vi "DisplayPanel.vi"() -> ()   [LabVIEW 2013]
uses:
  MvLVLib/MvCameraControl.lvlib
panel:
  in  "TimerTriggerActivation":u16(ring) items=["RisingEdge", "FallingEdge", "AnyEdge", "LevelHigh", "LevelLow"]
  in  "TimerTriggerSoftware":bool
  in  "TimerTriggerSource":u16(ring) items=["Off", "OptoCoupledInput0", "OptoCoupledInput1", "OptoCoupledInput2", "OptoCoupledInput3", "RS422diffInput0", "RS422diffInput1", "RS422diffInput2", "RS422diffInput3", "TTLInput0", "TTLInput1", "TTLInput2", "TTLInput3", "Timer0Active", "Timer1Active", "Timer2Active", "Timer3Active", "Encoder0", "Encoder1", "SoftwareSignal0", "Continuous"]
  in  "TimerFrequency":u32
  in  "TimerDelay":u32
  in  "TimerDuration":u32
  in  "TimerSelector":u16(ring) items=["Timer0", "Timer1", "Timer2", "Timer3"]
  in  "Interface List":u16(ring)
  out "handle":u64 format="%x"
  in  "Close Interface":bool
  in  "Open Interface":bool
  in  "Enum Interface":bool
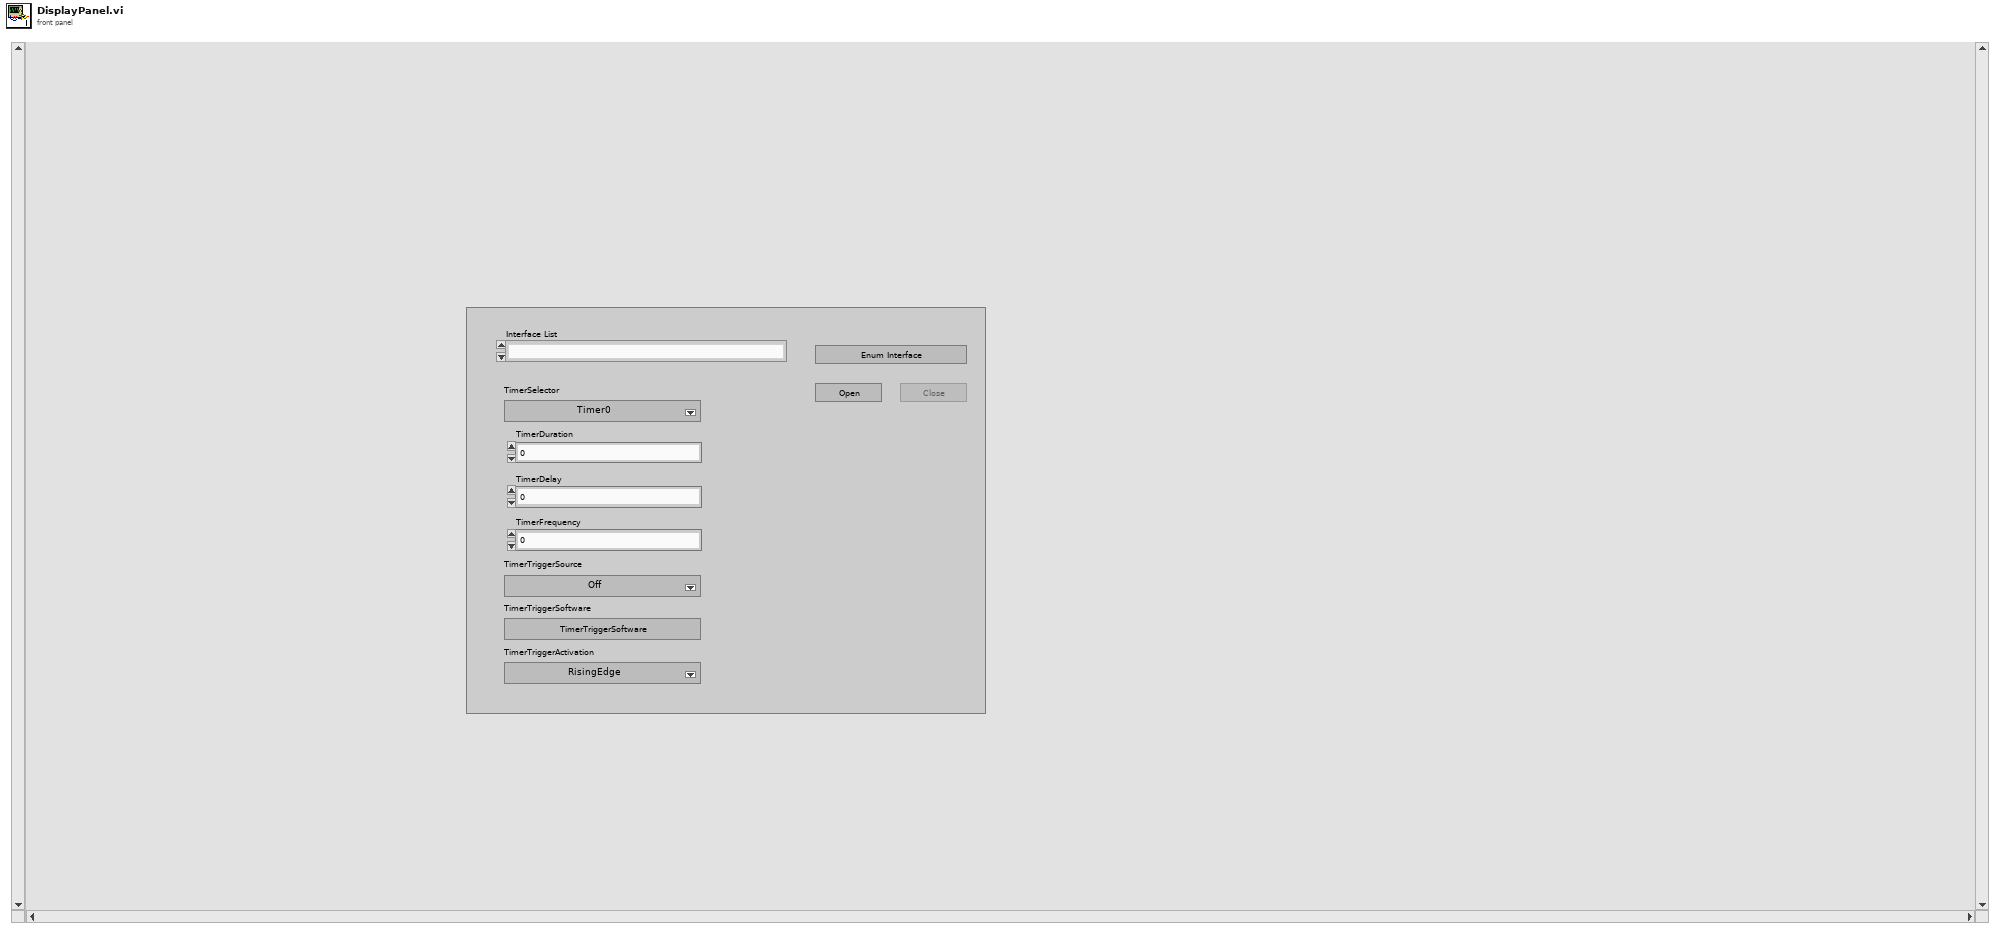
[diagram p1: front panel]
types:
  T1 = enum8{"Enabled", "Disabled", "Disabled and Grayed Out"}
  T2 = cluster{"nTLayerType":u32, "nPCIEInfo":u32, "chInterfaceID":string, "chDisplayName":string, "chSerialNumber":string, "chModelName":string, "chManufacturer":string, "chDeviceVersion":string, "chUserDefinedName":string}[]
  T3 = cluster{"nCurValue":u32, "nSupportedNum":u32, "nSupportValue":u32[], "nReserved[0]":u32, "nReserved[1]":u32, "nReserved[2]":u32, "nReserved[3]":u32}
  T4 = cluster{"nValue":u32, "chSymbolic":string, "nReserved[0]":u32, "nReserved[1]":u32, "nReserved[2]":u32, "nReserved[3]":u32}
  T5 = cluster{"nCurValue":u32, "nMax":u32, "nMin":u32, "nInc":u32, "nReserved[0]":u32, "nReserved[1]":u32, "nReserved[2]":u32, "nReserved[3]":u32}
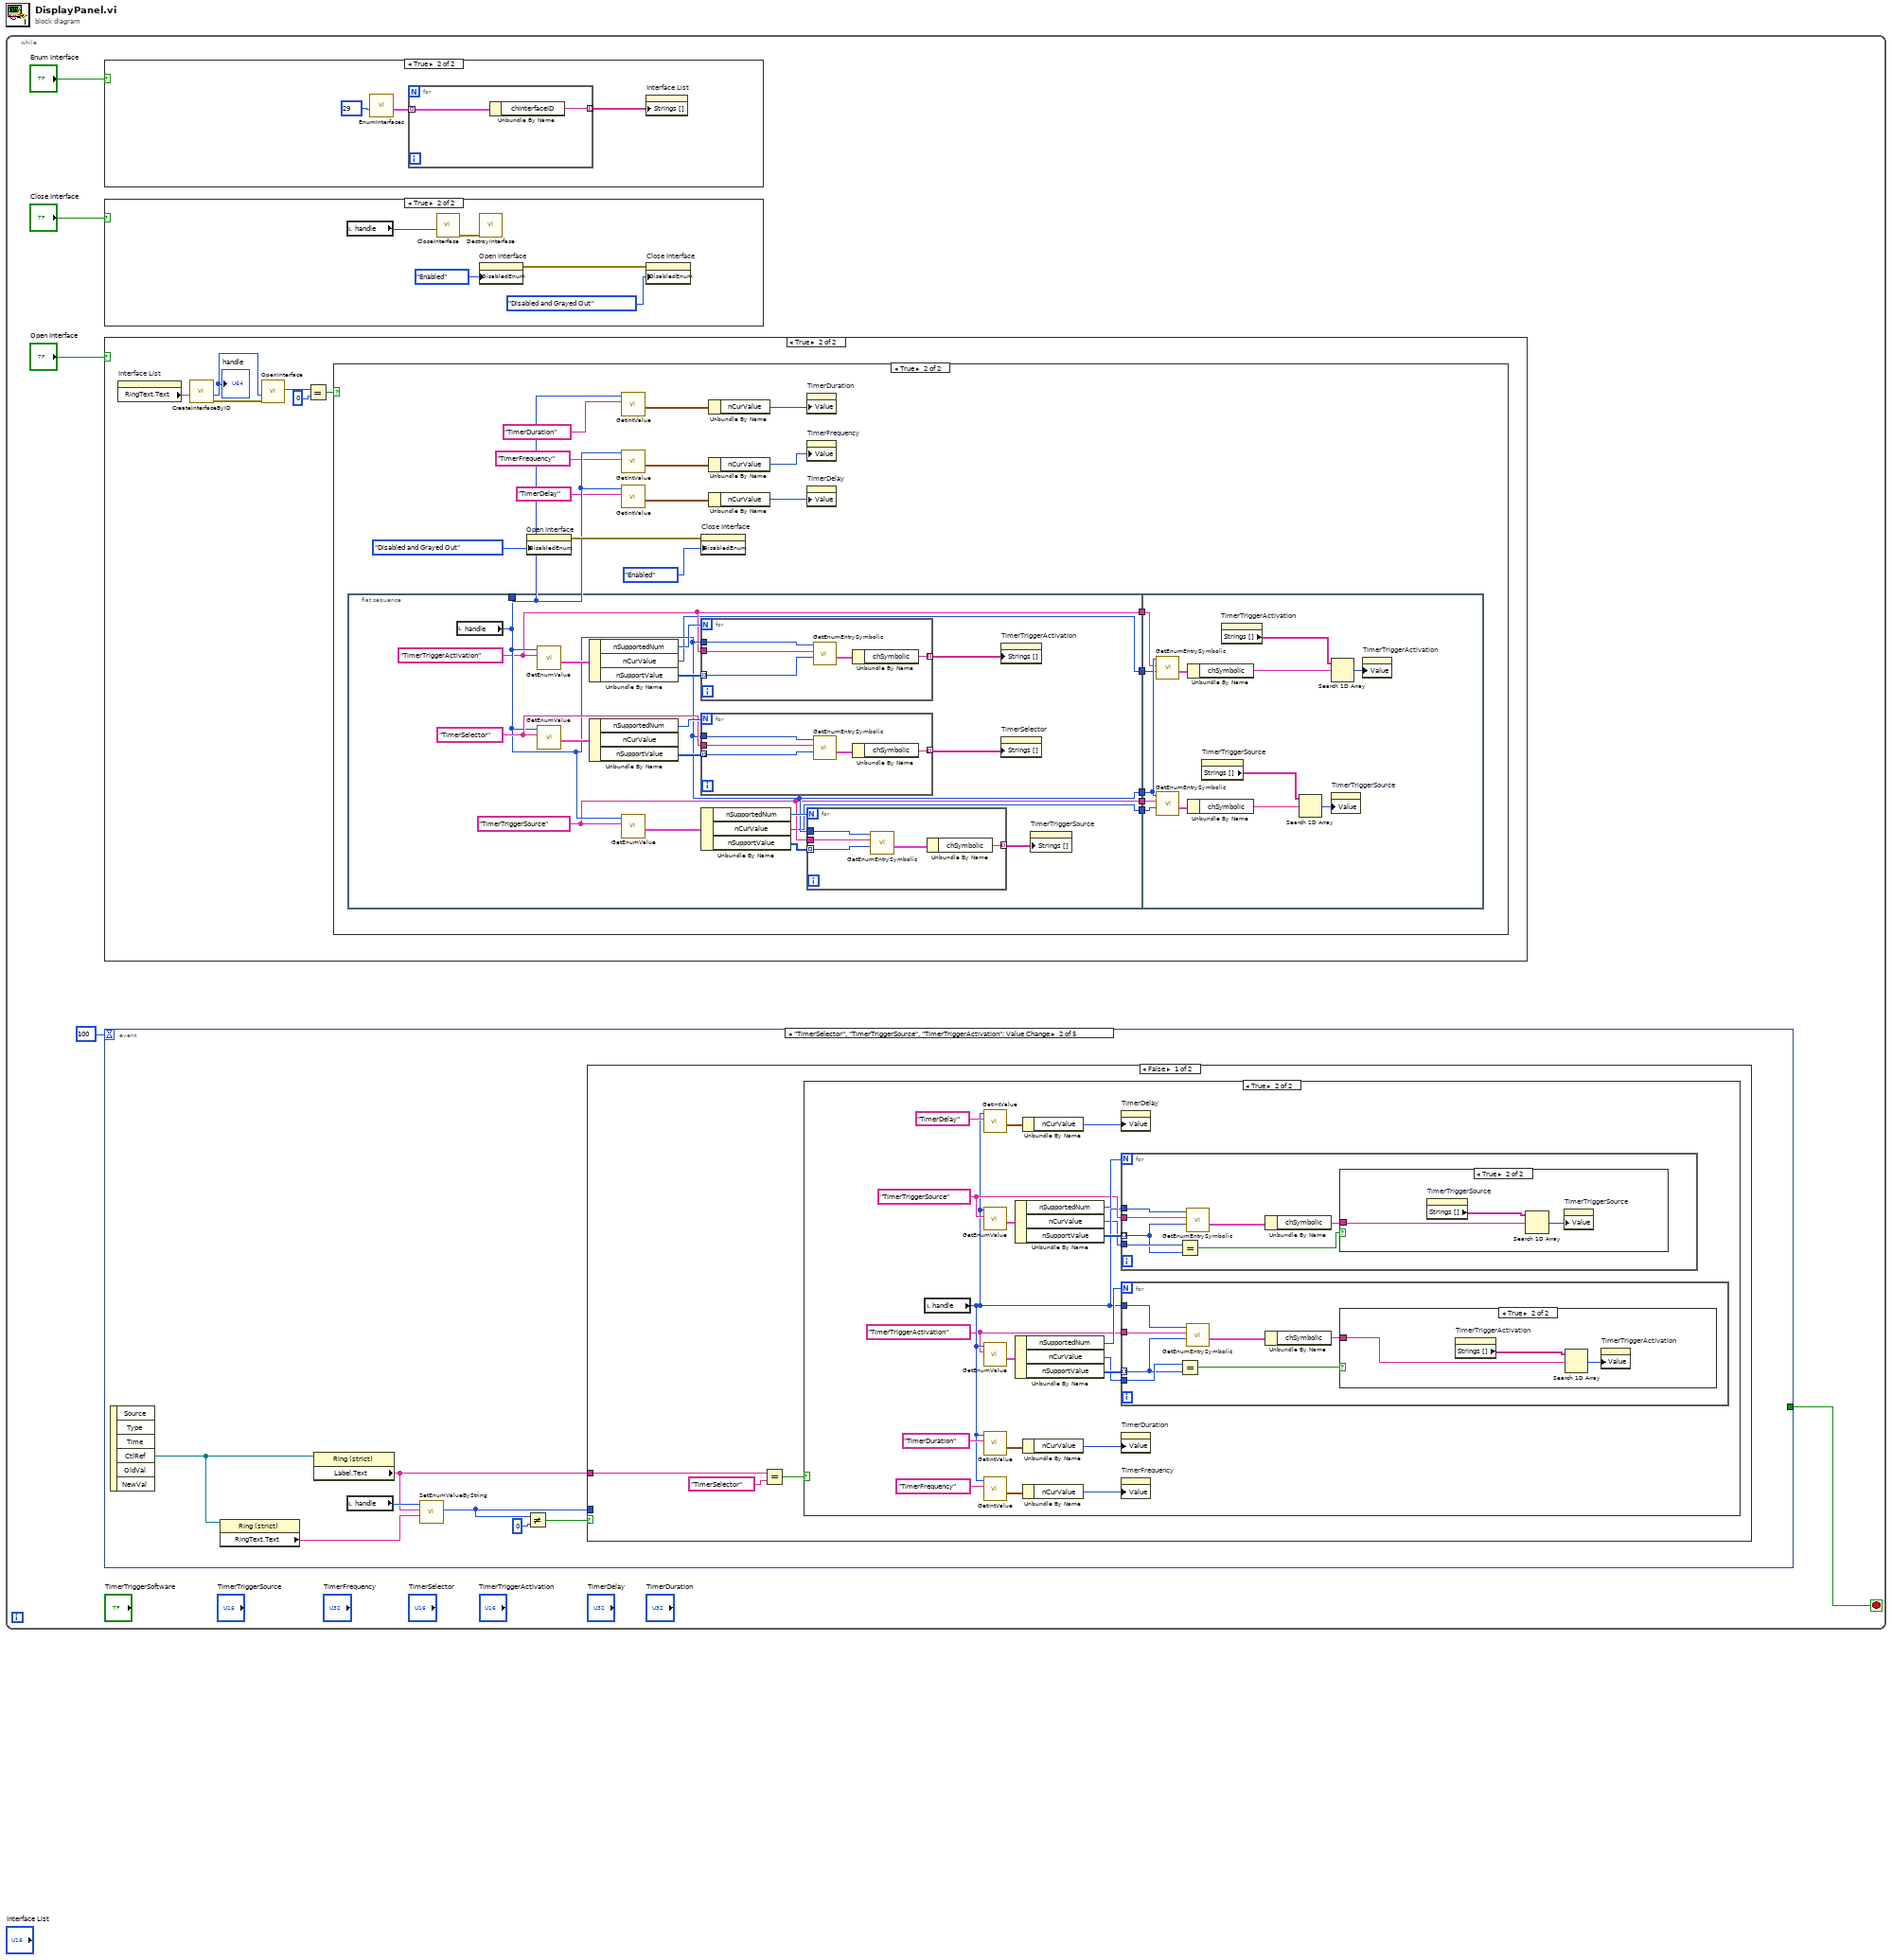
[diagram p0: block diagram]
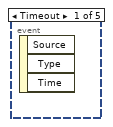
[diagram p2: hidden frame]
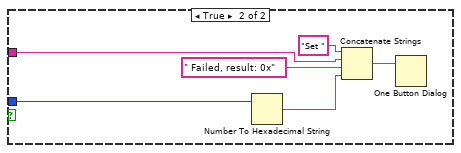
[diagram p6: hidden frame]
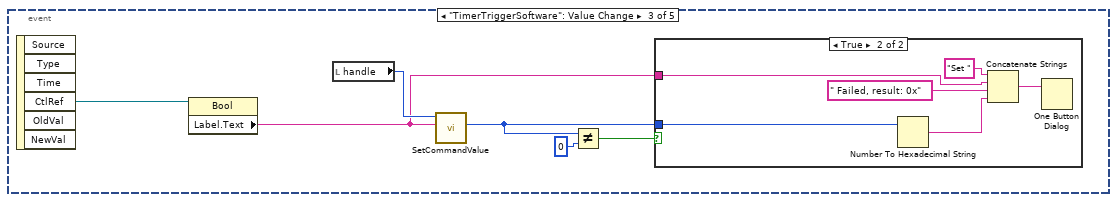
[diagram p7: hidden frame]
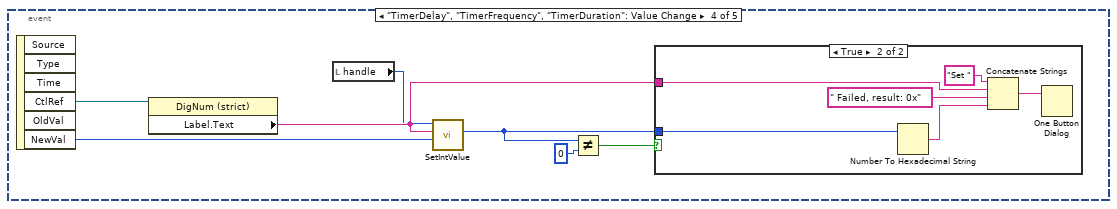
[diagram p9: hidden frame]
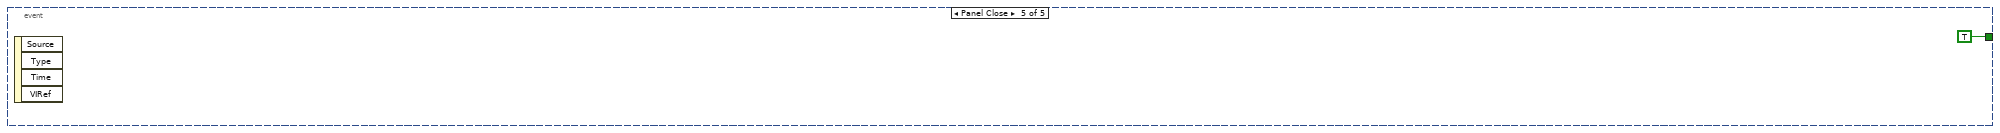
[diagram p11: hidden frame]
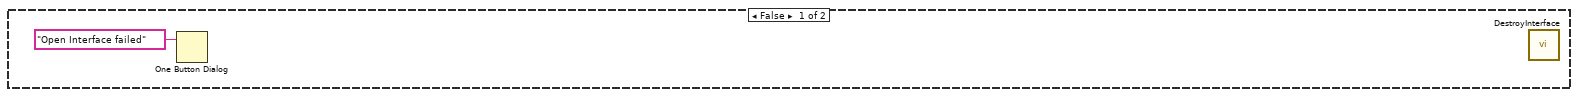
[diagram p14: hidden frame]
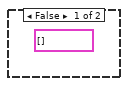
[diagram p15: hidden frame]
diagram:
  n1 = while {
    stop <- w2 stop-if-true
    n2 = case shown="True" "Enum Interface" {
      frame False {
        (unwired) T2 [] ("pInterfaceInfoList")
      }
      frame True {
        n3 = call "EnumInterfaces.vi"("nTLayerType"=u32 29) -> ("pInterfaceInfoList"=w164:T2)  [unwired: 8 in, 2 out]
        n4 = for {
          tunnel: w164 -> [w168] mode=indexing
          tunnel: [w167] -> w165 mode=indexing
          n5 = Unbundle By Name(w168) -> ("chInterfaceID"=w167:string)
        }
        n6 = property on="Interface List" class="Ring (strict)"("Strings []"=w165) -> ()  [unwired: 2 in, 2 out]
      }
    }
    n7 = case shown="True" "Close Interface" {
      frame False {
      }
      frame True {
        n8 = local read "handle"() -> (w89:u64)
        n9 = call "CloseInterface.vi"("handle"=w89) -> ("error out"=w92:errorcluster)  [unwired: 9 in, 1 out]
        n10 = call "DestroyInterface.vi"("error in (no error)"=w92) -> ()  [unwired: 9 in, 2 out]
        n11 = property on="Open Interface" class="Bool"("DisabledEnum"=T1."Enabled" ("Disabled")) -> (error out=w91:errorcluster)  [unwired: 2 in, 1 out]
        n12 = property on="Close Interface" class="Bool"(error in=w91, "DisabledEnum"=T1."Disabled and Grayed Out" ("Disabled")) -> ()  [unwired: 1 in, 2 out]
      }
    }
    n13 = case shown="True" "Open Interface" {
      frame False {
      }
      frame True {
        n14 = property on="Interface List" class="Ring (strict)"() -> ("RingText.Text"=w93:string)  [unwired: 2 in, 2 out]
        n15 = call "CreateInterfaceByID.vi"("pInterfaceID"=w93) -> ("error out"=w98:errorcluster, "handle"=w94:i64)  [unwired: 8 in, 1 out]
        "handle" <- w94
        n16 = call "OpenInterface.vi"("error in (no error)"=w98, "handle"=w94) -> ("return type"=w95:i32)  [unwired: 8 in, 1 out]
        n17 = Equal?(x=w95, y=u64 0) -> (x = y?=w96:bool)
        n18 = case shown="True" w96 {
          frame False {
            n19 = One Button Dialog(message="Open Interface failed") -> ()  [unwired: 1 in, 1 out]
            n20 = call "DestroyInterface.vi"() -> ()  [unwired: 10 in, 2 out]
          }
          frame True {
            n21 = flat-sequence {
              tunnel: [w122] -> w114
              tunnel: [w122] -> w104
              tunnel: [w121] -> w103
              tunnel: [w120] -> w102
              tunnel: [w119] -> w101
              tunnel: [w118] -> w100
              tunnel: w104 -> [w153]
              tunnel: w103 -> [w163]
              tunnel: w102 -> [w162]
              tunnel: w101 -> [w152]
              tunnel: w100 -> [w151]
              frame #0 {
                w119 = "TimerTriggerActivation" ("strKey")
                w121 = "TimerTriggerSource" ("strKey")
                w132 = "TimerSelector" ("strKey")
                n22 = local read "handle"() -> (w122:u64)
                n23 = call "GetEnumValue.vi"("strKey"=w119, "handle"=w122) -> ("pEnumValue out"=w125:T3)  [unwired: 6 in, 3 out]
                n24 = call "GetEnumValue.vi"("strKey"=w132, "handle"=w122) -> ("pEnumValue out"=w133:T3)  [unwired: 6 in, 3 out]
                n25 = Unbundle By Name(w125) -> ("nSupportedNum"=w123:u32, "nCurValue"=w118:u32, "nSupportValue"=w126:u32[])
                n26 = Unbundle By Name(w133) -> ("nSupportedNum"=w134:u32, "nSupportValue"=w131:u32[])  [unwired: 1 out]
                n27 = call "GetEnumValue.vi"("strKey"=w121, "handle"=w122) -> ("pEnumValue out"=w129:T3)  [unwired: 6 in, 3 out]
                n28 = for {
                  N: w123 -> [_]
                  tunnel: w119 -> [w140]
                  tunnel: [w138] -> w124 mode=indexing
                  tunnel: w126 -> [w137] mode=indexing
                  tunnel: w122 -> [w136]
                  n29 = call "GetEnumEntrySymbolic.vi"("nValue"=w137, "strKey"=w140, "handle"=w136) -> ("EnumEntry"=w139:T4)  [unwired: 5 in, 3 out]
                  n30 = Unbundle By Name(w139) -> ("chSymbolic"=w138:string)
                }
                n31 = for {
                  N: w134 -> [_]
                  tunnel: w132 -> [w150]
                  tunnel: w122 -> [w149]
                  tunnel: [w147] -> w135 mode=indexing
                  tunnel: w131 -> [w146] mode=indexing
                  n32 = call "GetEnumEntrySymbolic.vi"("nValue"=w146, "strKey"=w150, "handle"=w149) -> ("EnumEntry"=w148:T4)  [unwired: 5 in, 3 out]
                  n33 = Unbundle By Name(w148) -> ("chSymbolic"=w147:string)
                }
                n34 = Unbundle By Name(w129) -> ("nSupportedNum"=w127:u32, "nCurValue"=w120:u32, "nSupportValue"=w130:u32[])
                n35 = for {
                  N: w127 -> [_]
                  tunnel: w121 -> [w145]
                  tunnel: [w143] -> w128 mode=indexing
                  tunnel: w130 -> [w142] mode=indexing
                  tunnel: w122 -> [w141]
                  n36 = call "GetEnumEntrySymbolic.vi"("nValue"=w142, "strKey"=w145, "handle"=w141) -> ("EnumEntry"=w144:T4)  [unwired: 5 in, 3 out]
                  n37 = Unbundle By Name(w144) -> ("chSymbolic"=w143:string)
                }
                n38 = property on="TimerTriggerActivation" class="Ring (strict)"("Strings []"=w124) -> ()  [unwired: 2 in, 2 out]
                n39 = property on="TimerSelector" class="Ring (strict)"("Strings []"=w135) -> ()  [unwired: 2 in, 2 out]
                n40 = property on="TimerTriggerSource" class="Ring (strict)"("Strings []"=w128) -> ()  [unwired: 2 in, 2 out]
              }
              frame #1 {
                n41 = call "GetEnumEntrySymbolic.vi"("nValue"=w151, "strKey"=w152, "handle"=w153) -> ("EnumEntry"=w156:T4)  [unwired: 5 in, 3 out]
                n42 = call "GetEnumEntrySymbolic.vi"("nValue"=w162, "strKey"=w163, "handle"=w153) -> ("EnumEntry"=w159:T4)  [unwired: 5 in, 3 out]
                n43 = Unbundle By Name(w156) -> ("chSymbolic"=w157:string)
                n44 = Unbundle By Name(w159) -> ("chSymbolic"=w158:string)
                n45 = property on="TimerTriggerSource" class="Ring (strict)"() -> ("Strings []"=w160:string[])  [unwired: 2 in, 2 out]
                n46 = property on="TimerTriggerActivation" class="Ring (strict)"() -> ("Strings []"=w155:string[])  [unwired: 2 in, 2 out]
                n47 = Search 1D Array(1D array=w160, element=w158) -> (index of element=w161:i32)  [unwired: 1 in]
                n48 = Search 1D Array(1D array=w155, element=w157) -> (index of element=w154:i32)  [unwired: 1 in]
                n49 = property on="TimerTriggerSource" class="Ring (strict)"("Value"=w161) -> ()  [unwired: 2 in, 2 out]
                n50 = property on="TimerTriggerActivation" class="Ring (strict)"("Value"=w154) -> ()  [unwired: 2 in, 2 out]
              }
            }
            n51 = property on="Open Interface" class="Bool"("DisabledEnum"=T1."Disabled and Grayed Out" ("Disabled")) -> (error out=w116:errorcluster)  [unwired: 2 in, 1 out]
            n52 = call "GetIntValue.vi"("strKey"="TimerDuration", "handle"=w114) -> ("pIntValue out"=w112:T5)  [unwired: 6 in, 3 out]
            n53 = call "GetIntValue.vi"("strKey"="TimerFrequency", "handle"=w114) -> ("pIntValue out"=w106:T5)  [unwired: 6 in, 3 out]
            n54 = call "GetIntValue.vi"("strKey"="TimerDelay", "handle"=w114) -> ("pIntValue out"=w109:T5)  [unwired: 6 in, 3 out]
            n55 = property on="Close Interface" class="Bool"(error in=w116, "DisabledEnum"=T1."Enabled" ("Disabled")) -> ()  [unwired: 1 in, 2 out]
            n56 = Unbundle By Name(w112) -> ("nCurValue"=w111:u32)
            n57 = Unbundle By Name(w106) -> ("nCurValue"=w105:u32)
            n58 = Unbundle By Name(w109) -> ("nCurValue"=w110:u32)
            n59 = property on="TimerDuration" class="DigNum (strict)"("Value"=w111) -> ()  [unwired: 2 in, 2 out]
            n60 = property on="TimerFrequency" class="DigNum (strict)"("Value"=w105) -> ()  [unwired: 2 in, 2 out]
            n61 = property on="TimerDelay" class="DigNum (strict)"("Value"=w110) -> ()  [unwired: 2 in, 2 out]
          }
        }
      }
    }
    n62 = event shown="[1] \"TimerSelector\", \"TimerTriggerSource\", \"TimerTriggerActivation\": Value Change" {
      selector: _ -> [_ _ _ _ _]
      dyn-events: _ -> [_ _ _ _ _]
      timeout: 100 -> [_ _ _ _ _]
      tunnel: [_ _ _ _ TRUE] -> w2
      event Timeout {
        n63 = event-data() -> ()  [unwired: 1 in, 3 out]
      }
      event "TimerSelector", "TimerTriggerSource", "TimerTriggerActivation": Value Change {
        n64 = event-data() -> ("CtlRef"=w10:refnum<vi>)  [unwired: 1 in, 5 out]
        n65 = property class="Ring (strict)"(reference=w10) -> ("RingText.Text"=w11:string)  [unwired: 1 in, 2 out]
        n66 = property class="Ring (strict)"(reference=w10) -> ("Label.Text"=w7:string)  [unwired: 1 in, 2 out]
        n67 = local read "handle"() -> (w12:u64)
        n68 = call "SetEnumValueByString.vi"("strValue"=w11, "strKey"=w7, "handle"=w12) -> ("function return"=w6:i32)  [unwired: 6 in, 2 out]
        n69 = Not Equal?(x=w6, y=0) -> (x != y?=w8:bool)
        n70 = case shown="False" w8 {
          tunnel: w7 -> [w15 w60]
          tunnel: w6 -> [_ w59]
          frame False {
            n71 = Equal?(x=w15, y="TimerSelector") -> (x = y?=w13:bool)
            n72 = case shown="True" w13 {
              frame False {
              }
              frame True {
                w18 = "TimerTriggerActivation" ("strKey")
                w21 = "TimerTriggerSource" ("strKey")
                n73 = local read "handle"() -> (w19:u64)
                n74 = call "GetIntValue.vi"("strKey"="TimerDelay", "handle"=w19) -> ("pIntValue out"=w28:T5)  [unwired: 6 in, 3 out]
                n75 = call "GetEnumValue.vi"("strKey"=w21, "handle"=w19) -> ("pEnumValue out"=w22:T3)  [unwired: 6 in, 3 out]
                n76 = call "GetEnumValue.vi"("strKey"=w18, "handle"=w19) -> ("pEnumValue out"=w34:T3)  [unwired: 6 in, 3 out]
                n77 = call "GetIntValue.vi"("strKey"="TimerDuration", "handle"=w19) -> ("pIntValue out"=w25:T5)  [unwired: 6 in, 3 out]
                n78 = call "GetIntValue.vi"("strKey"="TimerFrequency", "handle"=w19) -> ("pIntValue out"=w31:T5)  [unwired: 6 in, 3 out]
                n79 = Unbundle By Name(w22) -> ("nSupportedNum"=w23:u32, "nCurValue"=w16:u32, "nSupportValue"=w20:u32[])
                n80 = Unbundle By Name(w34) -> ("nSupportedNum"=w35:u32, "nCurValue"=w17:u32, "nSupportValue"=w33:u32[])
                n81 = Unbundle By Name(w28) -> ("nCurValue"=w27:u32)
                n82 = Unbundle By Name(w25) -> ("nCurValue"=w26:u32)
                n83 = Unbundle By Name(w31) -> ("nCurValue"=w32:u32)
                n84 = property on="TimerDelay" class="DigNum (strict)"("Value"=w27) -> ()  [unwired: 2 in, 2 out]
                n85 = for {
                  N: w23 -> [_]
                  tunnel: w21 -> [w52]
                  tunnel: w19 -> [w51]
                  tunnel: w20 -> [w47] mode=indexing
                  tunnel: w16 -> [w48]
                  n86 = Equal?(x=w48, y=w47) -> (x = y?=w49:bool)
                  n87 = call "GetEnumEntrySymbolic.vi"("nValue"=w47, "strKey"=w52, "handle"=w51) -> ("EnumEntry"=w50:T4)  [unwired: 5 in, 3 out]
                  n88 = Unbundle By Name(w50) -> ("chSymbolic"=w46:string)
                  n89 = case shown="True" w49 {
                    tunnel: w46 -> [_ w54]
                    frame False {
                    }
                    frame True {
                      n90 = property on="TimerTriggerSource" class="Ring (strict)"() -> ("Strings []"=w55:string[])  [unwired: 2 in, 2 out]
                      n91 = Search 1D Array(1D array=w55, element=w54) -> (index of element=w53:i32)  [unwired: 1 in]
                      n92 = property on="TimerTriggerSource" class="Ring (strict)"("Value"=w53) -> ()  [unwired: 2 in, 2 out]
                    }
                  }
                }
                n93 = for {
                  N: w35 -> [_]
                  tunnel: w18 -> [w42]
                  tunnel: w19 -> [w41]
                  tunnel: w33 -> [w37] mode=indexing
                  tunnel: w17 -> [w38]
                  n94 = Equal?(x=w38, y=w37) -> (x = y?=w39:bool)
                  n95 = call "GetEnumEntrySymbolic.vi"("nValue"=w37, "strKey"=w42, "handle"=w41) -> ("EnumEntry"=w40:T4)  [unwired: 5 in, 3 out]
                  n96 = Unbundle By Name(w40) -> ("chSymbolic"=w36:string)
                  n97 = case shown="True" w39 {
                    tunnel: w36 -> [_ w43]
                    frame False {
                    }
                    frame True {
                      n98 = property on="TimerTriggerActivation" class="Ring (strict)"() -> ("Strings []"=w44:string[])  [unwired: 2 in, 2 out]
                      n99 = Search 1D Array(1D array=w44, element=w43) -> (index of element=w45:i32)  [unwired: 1 in]
                      n100 = property on="TimerTriggerActivation" class="Ring (strict)"("Value"=w45) -> ()  [unwired: 2 in, 2 out]
                    }
                  }
                }
                n101 = property on="TimerDuration" class="DigNum (strict)"("Value"=w26) -> ()  [unwired: 2 in, 2 out]
                n102 = property on="TimerFrequency" class="DigNum (strict)"("Value"=w32) -> ()  [unwired: 2 in, 2 out]
              }
            }
          }
          frame True {
            n103 = Number To Hexadecimal String(2:w59) -> (0:w57:string)  [unwired: 1 in]
            n104 = Concatenate Strings("Set " ("message"), w60, " Failed, result: 0x" ("string"), w57) -> (w56:string)
            n105 = One Button Dialog(message=w56) -> ()  [unwired: 1 in, 1 out]
          }
        }
      }
      event "TimerTriggerSoftware": Value Change {
        n106 = event-data() -> ("CtlRef"=w66:refnum<vi>)  [unwired: 1 in, 5 out]
        n107 = property class="Bool"(reference=w66) -> ("Label.Text"=w62:string)  [unwired: 1 in, 2 out]
        n108 = local read "handle"() -> (w65:u64)
        n109 = call "SetCommandValue.vi"("strValue"=w62, "handle"=w65) -> ("function return"=w63:i32)  [unwired: 7 in, 2 out]
        n110 = Not Equal?(x=w63, y=0) -> (x != y?=w67:bool)
        n111 = case shown="True" w67 {
          tunnel: w63 -> [_ w69]
          tunnel: w62 -> [_ w68]
          frame False {
          }
          frame True {
            n112 = Number To Hexadecimal String(2:w69) -> (0:w71:string)  [unwired: 1 in]
            n113 = Concatenate Strings("Set " ("message"), w68, " Failed, result: 0x" ("string"), w71) -> (w70:string)
            n114 = One Button Dialog(message=w70) -> ()  [unwired: 1 in, 1 out]
          }
        }
      }
      event "TimerDelay", "TimerFrequency", "TimerDuration": Value Change {
        n115 = event-data() -> ("CtlRef"=w75:refnum<vi>, "NewVal"=w74:u32)  [unwired: 1 in, 4 out]
        n116 = property class="DigNum (strict)"(reference=w75) -> ("Label.Text"=w80:string)  [unwired: 1 in, 2 out]
        n117 = local read "handle"() -> (w78:u64)
        n118 = call "SetIntValue.vi"("nValue"=w74, "strKey"=w80, "handle"=w78) -> ("function return"=w79:i32)  [unwired: 6 in, 2 out]
        n119 = Not Equal?(x=w79, y=0) -> (x != y?=w77:bool)
        n120 = case shown="True" w77 {
          tunnel: w79 -> [_ w82]
          tunnel: w80 -> [_ w81]
          frame False {
          }
          frame True {
            n121 = Number To Hexadecimal String(2:w82) -> (0:w84:string)  [unwired: 1 in]
            n122 = Concatenate Strings("Set " ("message"), w81, " Failed, result: 0x" ("string"), w84) -> (w83:string)
            n123 = One Button Dialog(message=w83) -> ()  [unwired: 1 in, 1 out]
          }
        }
      }
      event Panel Close {
        n124 = event-data() -> ()  [unwired: 1 in, 4 out]
      }
    }
  }
